vi "Write Caption.vi"(5 "Caption":string, 9 "Page in":refnum<class "Page.lvclass">) -> (3 "Page out":refnum<class "Page.lvclass">)   [LabVIEW 2014, in "Raspberry Pi Compatible Compiler for LabVIEW.lvlib" / "Page.lvclass"]
uses:
  Page.lvclass
  Page.lvclass/Page.ctl
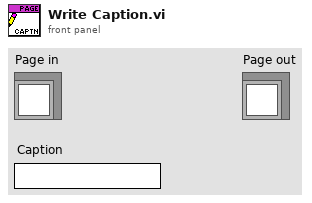
[diagram p1: front panel]
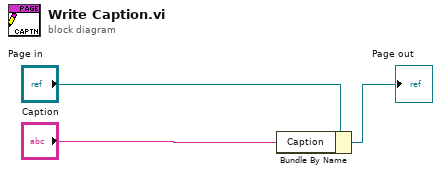
[diagram p0: block diagram]
diagram:
  n1 = Bundle By Name(cluster="Page in", "Caption"="Caption") -> (→"Page out":refnum<class "Page.lvclass">)
